vi "IsExistDataFrom1ListCtrl.vi"(11 "ArrayRef in":refnum<vi>) -> (2 "exist":bool, 3 "ArrayRef out":refnum<vi>)   [LabVIEW 2018, in "Library-Ctrl.lvlib"]
uses:
  Library-Ctrl.lvlib
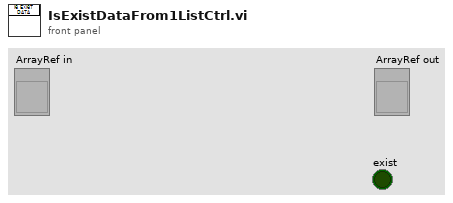
[diagram p1: front panel]
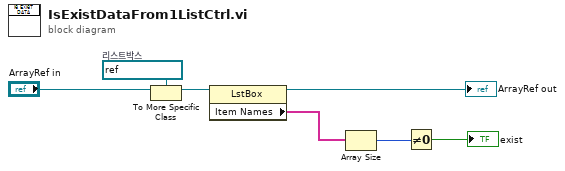
[diagram p0: block diagram]
diagram:
  w6 = refnum<vi> refnum  # 리스트박스
  n1 = To More Specific Class(target class=w6, reference="ArrayRef in") -> (specific class reference=w4:refnum<vi>)  [unwired: 1 in, 1 out]
  n2 = property class="LstBox"(reference=w4) -> (reference out=→"ArrayRef out":refnum<vi>, "Item Names"=w3:string[])  [unwired: 1 in, 1 out]
  n3 = Array Size(array=w3) -> (size(s)=w2:i32)
  n4 = Not Equal To 0?(x=w2) -> (x != 0?=→"exist":bool)
